vi "质控启动参数选择对话框.vi"(8 "COD":bool, 9 "总氮":bool, 10 "总磷":bool, 11 "氨氮":bool) -> (1 "取消启动":bool, 2 "确定启动":bool, 3 "启动模块":T1)   [LabVIEW 2016, in "质控单元.lvlib"]
panel:
  in  "CODCr":bool
  in  "总氮":bool
  in  "确定":bool
  in  "CODMn":bool
  in  "总磷":bool
  in  "取消":bool
  in  "氨氮":bool
  # "请选择加标回收模块"
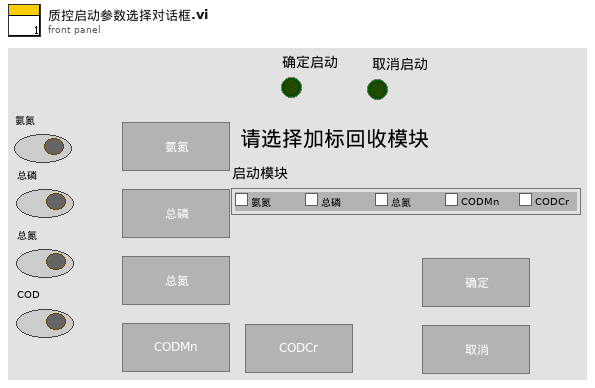
[diagram p1: front panel]
types:
  T1 = cluster{"氨氮":bool, "总磷":bool, "总氮":bool, "CODMn":bool, "CODCr":bool}
  T2 = enum8{"Enabled", "Disabled", "Disabled and Grayed Out"}
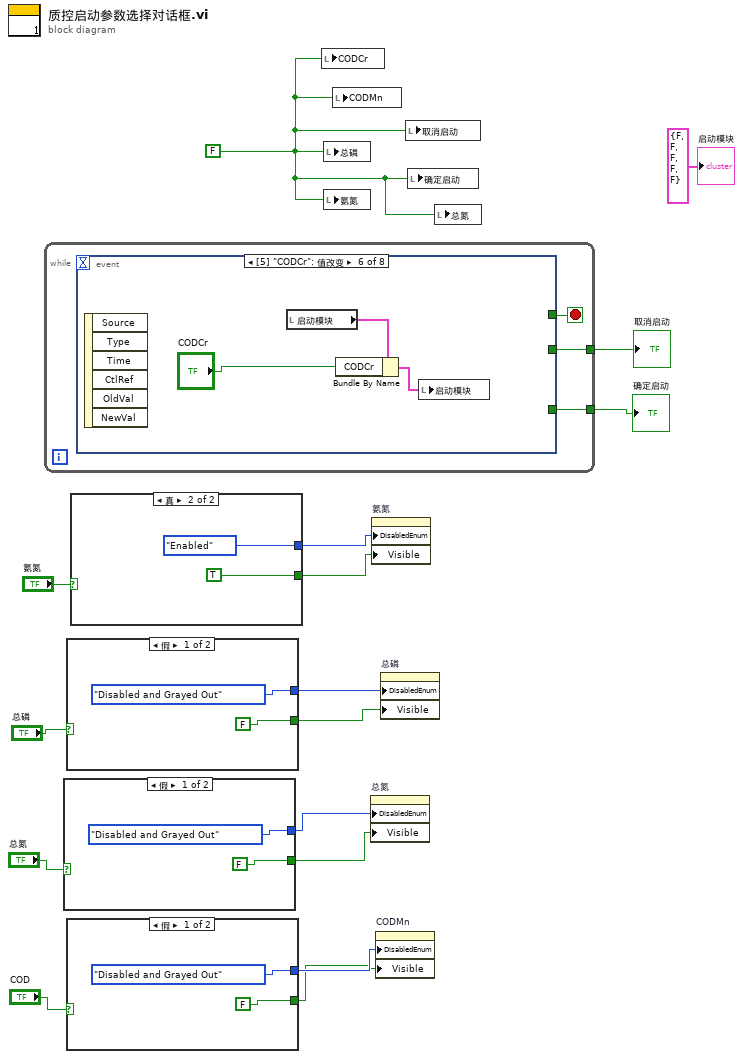
[diagram p0: block diagram]
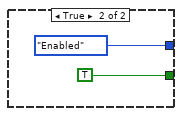
[diagram p2: hidden frame]
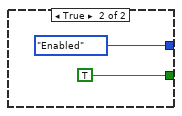
[diagram p3: hidden frame]
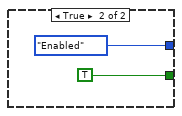
[diagram p4: hidden frame]
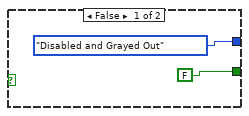
[diagram p5: hidden frame]
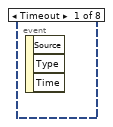
[diagram p6: hidden frame]
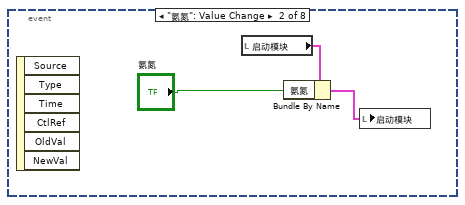
[diagram p7: hidden frame]
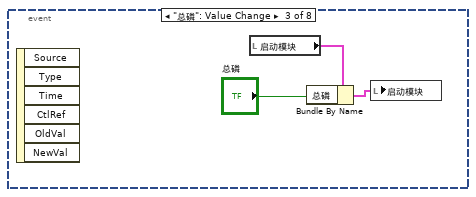
[diagram p8: hidden frame]
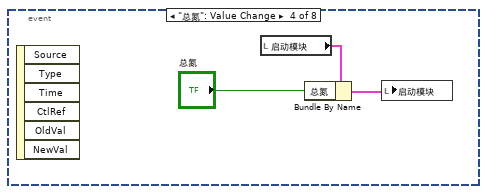
[diagram p9: hidden frame]
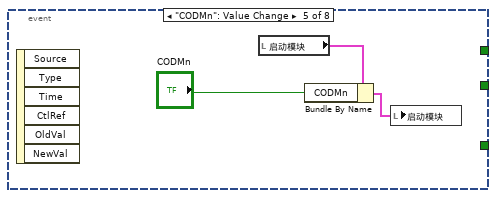
[diagram p10: hidden frame]
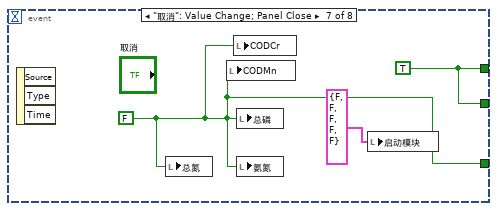
[diagram p11: hidden frame]
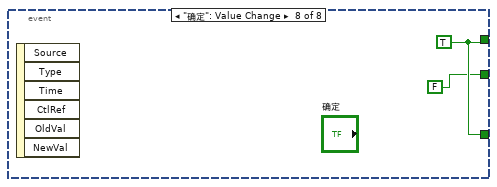
[diagram p12: hidden frame]
diagram:
  w1 = FALSE ("确定")
  n1 = while {
    tunnel: [w18] -> w16
    tunnel: [w17] -> w15
    stop <- w19 stop-if-true
    n2 = event shown="[5] \"CODCr\": 值改变" {
      selector: _ -> [_ _ _ _ _ _ _ _]
      dyn-events: _ -> [_ _ _ _ _ _ _ _]
      timeout: _ -> [_ _ _ _ _ _ _ _]
      tunnel: [_ _ _ _ _ _ w37 w39] -> w19
      tunnel: [_ _ _ _ _ _ w36 w39] -> w18
      tunnel: [_ _ _ _ _ _ w37 FALSE ("确定")] -> w17
      event Timeout {
        n3 = event-data() -> ()  [unwired: 1 in, 3 out]
      }
      event "氨氮": Value Change {
        n4 = event-data() -> ()  [unwired: 1 in, 6 out]
        n5 = local read "启动模块"() -> (w21:T1)
        n6 = Bundle By Name(cluster=w21, "氨氮"="氨氮") -> (w20:T1)
        n7 = local write "启动模块"(w20) -> ()
      }
      event "总磷": Value Change {
        n8 = event-data() -> ()  [unwired: 1 in, 6 out]
        n9 = local read "启动模块"() -> (w24:T1)
        n10 = Bundle By Name(cluster=w24, "总磷"="总磷") -> (w23:T1)
        n11 = local write "启动模块"(w23) -> ()
      }
      event "总氮": Value Change {
        n12 = event-data() -> ()  [unwired: 1 in, 6 out]
        n13 = local read "启动模块"() -> (w27:T1)
        n14 = Bundle By Name(cluster=w27, "总氮"="总氮") -> (w26:T1)
        n15 = local write "启动模块"(w26) -> ()
      }
      event "CODMn": Value Change {
        n16 = event-data() -> ()  [unwired: 1 in, 6 out]
        n17 = local read "启动模块"() -> (w30:T1)
        n18 = Bundle By Name(cluster=w30, "CODMn"="CODMn") -> (w29:T1)
        n19 = local write "启动模块"(w29) -> ()
      }
      event "CODCr": Value Change {
        n20 = event-data() -> ()  [unwired: 1 in, 6 out]
        n21 = local read "启动模块"() -> (w34:T1)
        n22 = Bundle By Name(cluster=w34, "CODCr"="CODCr") -> (w33:T1)
        n23 = local write "启动模块"(w33) -> ()
      }
      event "取消": Value Change; Panel Close {
        w36 = FALSE ("确定")
        w37 = TRUE ("确定")
        n24 = event-data() -> ()  [unwired: 1 in, 3 out]
        n25 = local write "总氮"(w36) -> ()
        n26 = local write "CODMn"(w36) -> ()
        n27 = local write "CODCr"(w36) -> ()
        n28 = local write "总磷"(w36) -> ()
        n29 = local write "氨氮"(w36) -> ()
        n30 = local write "启动模块"(T1 {"氨氮"=FALSE, "总磷"=FALSE, "总氮"=FALSE, "CODMn"=FALSE, "CODCr"=FALSE} ("启动模块")) -> ()
      }
      event "确定": Value Change {
        w39 = TRUE ("确定")
        n31 = event-data() -> ()  [unwired: 1 in, 6 out]
      }
    }
  }
  "确定启动" <- w16
  "取消启动" <- w15
  n32 = case shown="假" "总氮" {
    tunnel: [T2."Disabled and Grayed Out" ("禁用") T2."Enabled" ("禁用")] -> w6
    tunnel: [FALSE ("可见") TRUE ("可见")] -> w5
    frame False {
    }
    frame True {
    }
  }
  n33 = case shown="假" "总磷" {
    tunnel: [T2."Disabled and Grayed Out" ("禁用") T2."Enabled" ("禁用")] -> w8
    tunnel: [FALSE ("可见") TRUE ("可见")] -> w7
    frame False {
    }
    frame True {
    }
  }
  n34 = case shown="假" "COD" {
    tunnel: [T2."Disabled and Grayed Out" ("禁用") T2."Enabled" ("禁用")] -> w4
    tunnel: [FALSE ("可见") TRUE ("可见")] -> w3
    frame False {
    }
    frame True {
    }
  }
  n35 = case shown="真" "氨氮" {
    tunnel: [T2."Disabled and Grayed Out" ("禁用") T2."Enabled" ("禁用")] -> w10
    tunnel: [FALSE ("可见") TRUE ("可见")] -> w9
    frame False {
    }
    frame True {
    }
  }
  n36 = local write "CODCr"(w1) -> ()
  n37 = local write "总磷"(w1) -> ()
  n38 = local write "氨氮"(w1) -> ()
  n39 = local write "CODMn"(w1) -> ()
  n40 = property on="总氮" class="Bool (严格)"("DisabledEnum"=w6, "Visible"=w5) -> ()  [unwired: 2 in, 2 out]
  n41 = property on="氨氮" class="Bool (严格)"("DisabledEnum"=w10, "Visible"=w9) -> ()  [unwired: 2 in, 2 out]
  n42 = property on="CODMn" class="Bool (严格)"("DisabledEnum"=w4, "Visible"=w3) -> ()  [unwired: 2 in, 2 out]
  n43 = property on="总磷" class="Bool (严格)"("DisabledEnum"=w8, "Visible"=w7) -> ()  [unwired: 2 in, 2 out]
  n44 = local write "取消启动"(w1) -> ()
  n45 = local write "确定启动"(w1) -> ()
  n46 = local write "总氮"(w1) -> ()
  "启动模块" <- T1 {"氨氮"=FALSE, "总磷"=FALSE, "总氮"=FALSE, "CODMn"=FALSE, "CODCr"=FALSE} ("启动模块")
